vi "Entry.vi"(8 "error in (no error)":errorcluster, 11 "New State":refnum<class "IDLE.lvclass">) -> (0 "error out":errorcluster, 3 "State out":refnum<class "IDLE.lvclass">)   [LabVIEW 2024, in "Chef States.lvlib" / "IDLE.lvclass"]
doc: "This is an abstract method. Override this method to define the behavior when you enter the state."
uses:
  IDLE.lvclass
  <vilib>/ActorFramework/Actor/Actor.lvclass/Actor.ctl
  Root Actor Logic/Root Actor Logic Messages/Update State String Msg/Update State String Msg.lvclass/Update State String Msg.ctl
  <vilib>/ActorFramework/Message Enqueuer/Message Enqueuer.lvclass/Message Enqueuer.ctl
  <vilib>/ActorFramework/Message Enqueuer/Enqueue.vi
  Root Actor Logic/Root Actor Logic Messages/Update State String Msg/Update State String Msg.lvclass
  <vilib>/ActorFramework/Message Priority Queue/Priority Enqueue.vi
  Chef State/Chef State.lvclass
  IDLE.lvclass/IDLE.ctl
  <vilib>/ActorFramework/Actor/Actor.lvclass
  Timer Actor/Timer Actor Messages/Start Count Down Msg/Start Count Down Msg.lvclass
  C:/Users/burakkorkmaz/Desktop/Leveling/repo/Chef States/Chef State/Chef State.lvclass
  C:/Program Files/National Instruments/LabVIEW 2024/vi.lib/NI/Actors/State Actor/State Actor/State Actor.lvclass
  C:/Program Files/National Instruments/LabVIEW 2024/vi.lib/ActorFramework/Actor/Actor.lvclass
  C:/Users/burakkorkmaz/Desktop/Leveling/repo/Chef States Logic/Chef States Logic/Chef States Logic.lvclass
  C:/Users/burakkorkmaz/Desktop/Leveling/repo/Chef States/IDLE/IDLE.lvclass
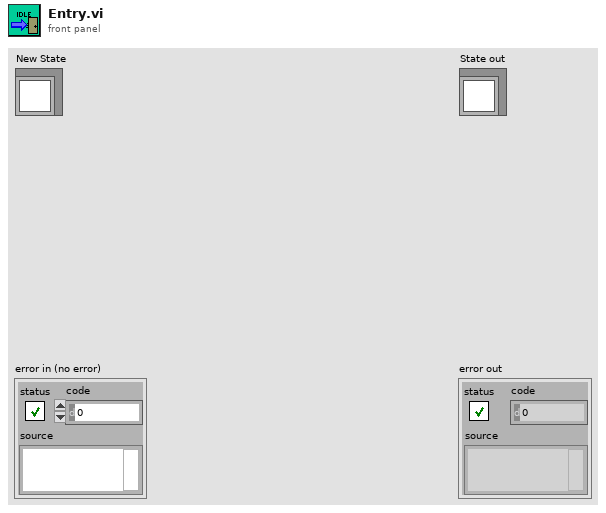
[diagram p1: front panel]
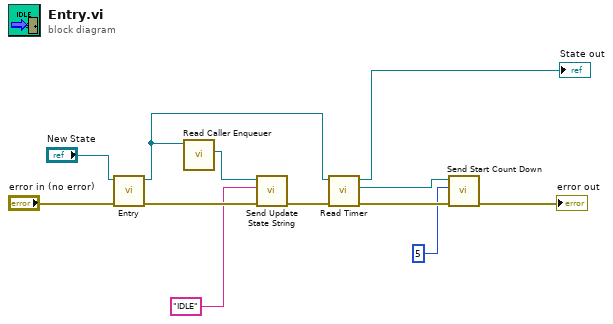
[diagram p0: block diagram]
diagram:
  n1 = call-parent "Entry.vi"("error in (no error)"="error in (no error)", "New State"="New State") -> ("error out"=w12:errorcluster, "State out"=w3:refnum<class "IDLE.lvclass">)  [unwired: 8 in]
  n2 = call <vilib>:"Read Caller Enqueuer.vi"("Actor"=w3) -> ("Caller Enqueuer"=w8:refnum<class "Message Enqueuer.lvclass">)  [unwired: 10 in]
  n3 = call "Send Update State String.vi"("error in (no error)"=w12, "State"="IDLE", "Message Enqueuer"=w8) -> ("error out"=w9:errorcluster)  [unwired: 7 in, 1 out]
  n4 = call-dynamic "Read Timer.vi"("error in (no error)"=w9, "Chef State in"=w3) -> ("error out"=w6:errorcluster, "Actor Framework:Message Enqueuer"=w4:refnum<class "Message Enqueuer.lvclass">, "Chef State out"=→"State out":refnum<class "IDLE.lvclass">)  [unwired: 7 in]
  n5 = call "Send Start Count Down.vi"("error in (no error)"=w6, "Seconds To Wait"=5, "Message Enqueuer"=w4) -> ("error out"=→"error out":errorcluster)  [unwired: 7 in, 1 out]
